vi "get child tag.vi"(0 "ChannalConfig":refnum<vi>, 11 "error in (no error)":errorcluster) -> (4 "ChannalConfig out":refnum<vi>, 6 "? parent":bool, 8 "tag and parent tag":cluster{"Tag":string, "Parent tag":string}, 10 "child tag":string[](array[string]), 15 "error out":errorcluster)   [LabVIEW 2011]
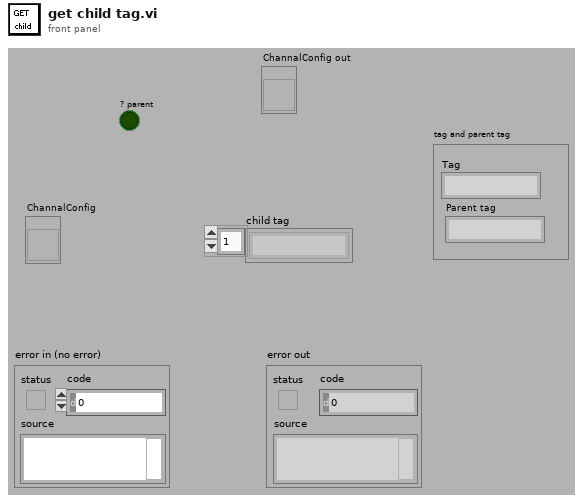
[diagram p1: front panel]
types:
  T1 = cluster{"Active Item Tag":string, "Navigate Tree:Get Child":string}
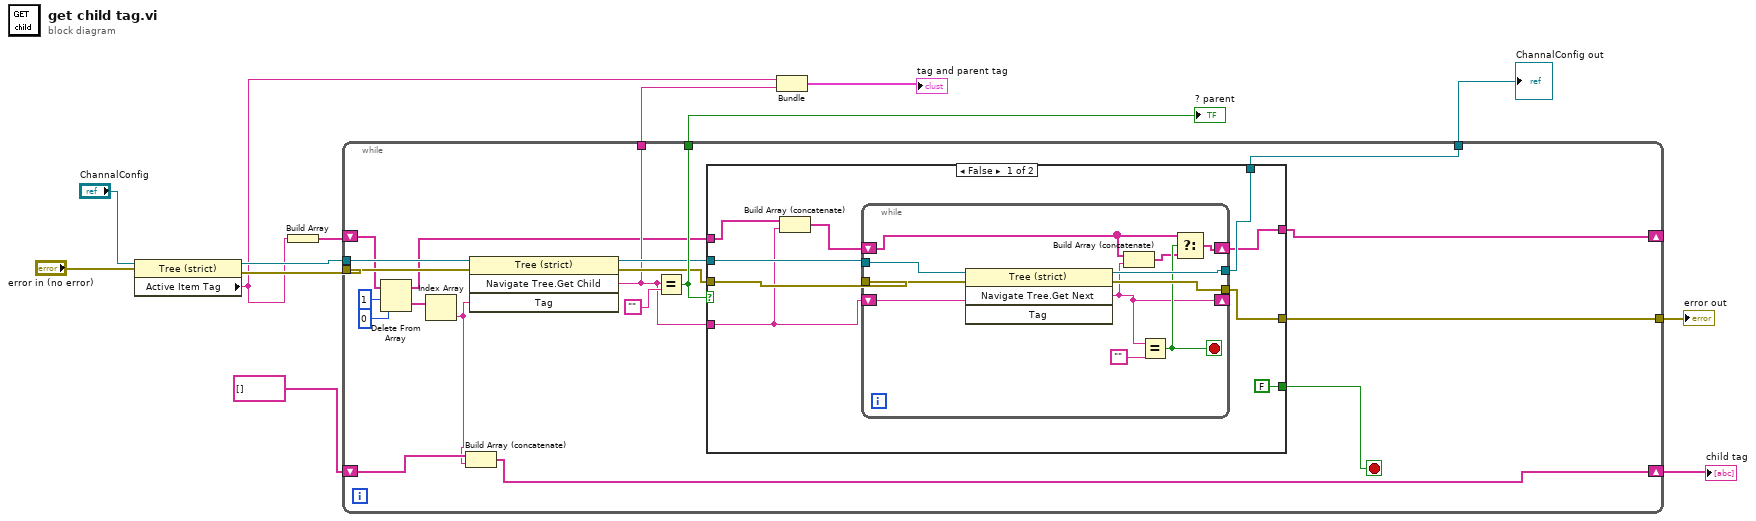
[diagram p0: block diagram]
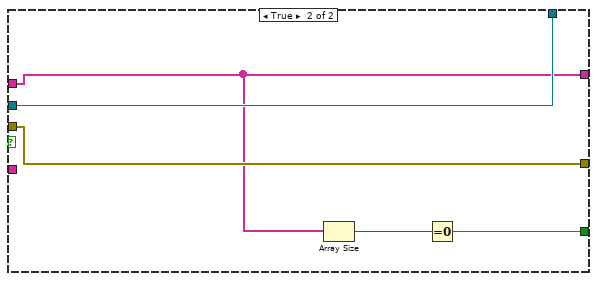
[diagram p2: hidden frame]
diagram:
  n1 = property class="Tree (strict)"(reference="ChannalConfig", error in="error in (no error)") -> (reference out=w13:refnum<vi>, error out=w9:errorcluster, "Active Item Tag"=w4:string)
  n2 = Build Array(w4) -> (w3:string[])
  n3 = while {
    tunnel: w13 -> [w32]
    tunnel: [w30] -> w12
    tunnel: [w28] -> w11
    tunnel: w9 -> [w27]
    tunnel: [w25] -> w8
    tunnel: [w24] -> w5
    shift-right: [w18] -> _
    shift-left: w3 -> [w21]
    shift-right: [w14] -> w1
    shift-left: string[] [] -> [w16]
    stop <- w17 stop-if-true
    n4 = Delete From Array(array=w21, length=1, index=0) -> (deleted portion=w19:string[], array with subset deleted=w20:string[])
    n5 = Index Array(array=w19) -> (element=w15:string)  [unwired: 1 in]
    n6 = Build Array (concatenate)(w16, w15) -> (w14:string[])
    n7 = invoke class="Tree (strict)" method="Navigate Tree.Get Child"(reference=w32, error in=w27, "Tag"=w15) -> (reference out=w29:refnum<vi>, error out=w26:errorcluster, "Navigate Tree:Get Child"=w24:string)  [unwired: 1 in, 1 out]
    n8 = Equal?(x=w24, y="") -> (x = y?=w30:bool)
    n9 = case shown="False" w30 {
      tunnel: w29 -> [w39 w57]
      tunnel: w24 -> [w36 _]
      tunnel: [w41 w57] -> w28
      tunnel: w26 -> [w38 w56]
      tunnel: [w40 w56] -> w25
      tunnel: [w34 w55] -> w18
      tunnel: w20 -> [w37 w55]
      tunnel: [FALSE w53] -> w17
      frame False {
        n10 = Build Array (concatenate)(w37, w36) -> (w35:string[])
        n11 = while {
          tunnel: w39 -> [w52]
          shift-right: [w44] -> _
          shift-left: w36 -> [w51]
          tunnel: [w49] -> w41
          tunnel: w38 -> [w48]
          tunnel: [w47] -> w40
          shift-right: [w42] -> w34
          shift-left: w35 -> [w45]
          stop <- w46 stop-if-true
          n12 = invoke class="Tree (strict)" method="Navigate Tree.Get Next"(reference=w52, error in=w48, "Tag"=w51) -> (reference out=w49:refnum<vi>, error out=w47:errorcluster, "Navigate Tree:Get Next Item"=w44:string)  [unwired: 1 in, 1 out]
          n13 = Build Array (concatenate)(w45, w44) -> (w43:string[])
          n14 = Equal?(x=w44, y="") -> (x = y?=w46:bool)
          n15 = Select(t=w45, s=w46, f=w43) -> (s? t:f=w42:string[])
        }
      }
      frame True {
        n16 = Array Size(array=w55) -> (size(s)=w54:i32)
        n17 = Equal To 0?(x=w54) -> (x = 0?=w53:bool)
      }
    }
  }
  "? parent" <- w12
  "ChannalConfig out" <- w11
  "error out" <- w8
  "child tag" <- w1
  n18 = Bundle("Active Item Tag"=w4, "Navigate Tree:Get Child"=w5) -> (→"tag and parent tag":T1)  [unwired: 1 out]
